vi "Configure Operation Mode.vi"(8 "error in (no error)":errorcluster, 10 "Operation Mode (0: OFF)":i32(ring) items=["OFF", "Parallel", "Series"], 11 "VISA resource name":refnum<visa-resource-name>) -> (0 "error out":errorcluster, 3 "VISA resource name out":refnum<visa-resource-name>)   [LabVIEW 2020, in "Keysight E36300 Series.lvlib"]
doc: "Configures power supply's operation mode.\n\n<b>Notes:</b>\nThis VI is not supported by EDU36311A model."
uses:
  Keysight E36300 Series.lvlib
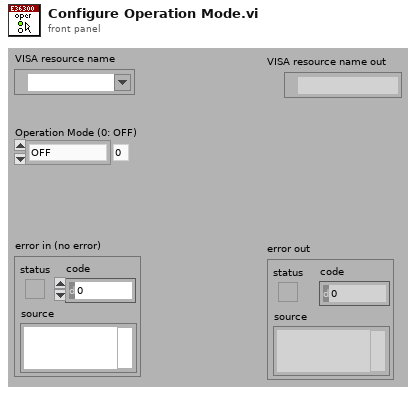
[diagram p1: front panel]
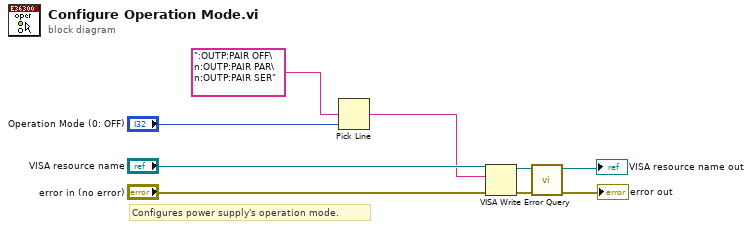
[diagram p0: block diagram]
diagram:
  # "Configures power supply's operation mode."
  n1 = Pick Line(multi-line string=":OUTP:PAIR OFF\n:OUTP:PAIR PAR\n:OUTP:PAIR SER", line index="Operation Mode (0: OFF)") -> (output string=w5:string)  [unwired: 1 in]
  n2 = VISA Write(VISA resource name="VISA resource name", write buffer=w5, error in (no error)="error in (no error)") -> (VISA resource name out=w4:refnum<visa-resource-name>, error out=w3:errorcluster)  [unwired: 1 out]
  n3 = call "Error Query.vi"("error in (no error)"=w3, "VISA resource name"=w4) -> ("error out"=→"error out":errorcluster, "VISA resource name out"=→"VISA resource name out":refnum<visa-resource-name>)  [unwired: 6 in, 2 out]
